vi "GPIO Read Value.vi"(7 "GPIO #":T1=-1, 8 "error in (no error)":errorcluster, 11 "FirmwareComms in":refnum<class "VisaComms.lvclass">) -> (0 "error out":errorcluster, 2 "Value":bool, 3 "FirmwareComms out":refnum<class "VisaComms.lvclass">)   [LabVIEW 2020, in "CTI.lvlib" / "VisaComms.lvclass"]
uses:
  VisaComms.lvclass
  GPIO Number.ctl
  VisaComms.lvclass/VisaComms.ctl
  CTI.lvlib
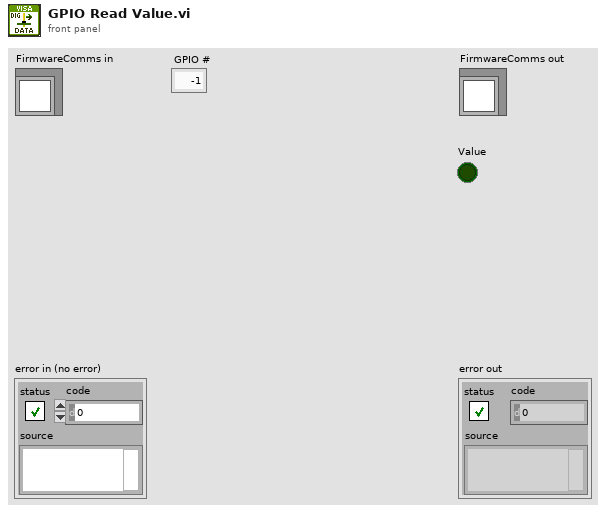
[diagram p1: front panel]
types:
  T1 = typedef "CTI.lvlib/GPIO Number.ctl" = i8
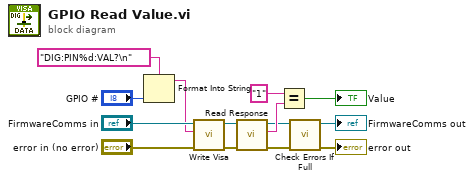
[diagram p0: block diagram]
diagram:
  n1 = Format Into String(format string="DIG:PIN%d:VAL?\n", "GPIO #") -> (resulting string=w11:string)  [unwired: 2 in, 1 out]
  n2 = call "Write Visa.vi"("error in (no error)"="error in (no error)", "write buffer"=w11, "VisaComms in"="FirmwareComms in") -> ("error out"=w9:errorcluster, "VisaComms out"=w7:refnum<class "VisaComms.lvclass">)  [unwired: 6 in, 1 out]
  n3 = call "Read Response.vi"("error in (no error)"=w9, "VisaComms in"=w7) -> ("error out"=w8:errorcluster, "Response"=w5:string, "VisaComms out"=w2:refnum<class "VisaComms.lvclass">)  [unwired: 7 in]
  n4 = Equal?(x="1", y=w5) -> (x = y?=→"Value":bool)
  n5 = call "Check Errors If Full.vi"("error in (no error)"=w8, "VisaComms in"=w2) -> ("error out"=→"error out":errorcluster, "VisaComms out"=→"FirmwareComms out":refnum<class "VisaComms.lvclass">)  [unwired: 8 in]
